vi "Pockels-Voltage limiter.vi"(1 "Pockels AO data in":dbl[](array[numeric])) -> (0 "Pockels AO data out":dbl[](array[numeric]))   [LabVIEW 2013]
uses:
  Globals/gl_Pockels control globals.vi
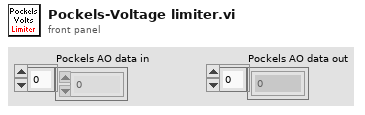
[diagram p1: front panel]
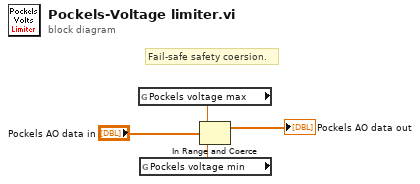
[diagram p0: block diagram]
diagram:
  # "Fail-safe safety coersion."
  n1 = global read "gl_Pockels control globals.vi" "Pockels voltage max"() -> (w2:dbl)
  n2 = global read "gl_Pockels control globals.vi" "Pockels voltage min"() -> (w1:dbl)
  n3 = In Range and Coerce(upper limit=w2, x="Pockels AO data in", lower limit=w1) -> (coerced(x)=→"Pockels AO data out":dbl[])  [unwired: 1 out]
